vi "niScope EX Multi-Device Configured Acquisition (TClk).vi"() -> ()   [LabVIEW 2013]
doc: "Example: TClk Synchronized Configured Acquisition\n\nRecommended Input Signal: 100 kHz, 4 Vpp, sine wave\n\nDevices Supported: Refer to NI Example Finder\n\nDescription:\n\nThis example configures all the digitizer's vertical, horizontal, and triggering properties before every acquisition. It allows you to experiment with numerous configurations, including acquisition types and triggering modes, since it supports nearly the entire functionality of NI-SCOPE.\n\nThis example also demonstrates how to easily synchronize an arbitrary number of digitizers with niTClk. The niTClk Configure for Homogeneous Triggers, niTClk Synchronize, and niTClk Initiate VIs make this very simple to accomplish. niTClk is useful when synchronized sampling and subsample trigger position are desired. Please refer to the niTClk documentation for more information.\n\nMany parameters are included on the front panel of this example. Notice the \"min sample rate\" compared to the \"actual sample rate,\" and similarly the \"min record length\" to the \"actual record length.\" The \"min\" values are specified with the Configure Horizontal Timing VI. NI-SCOPE maintains a constant time per record for each acquisition. So when you specify a min sample rate and a min record length, this determines the amount of time the acquisition should take:\n\n time per record = min record length / min sampling rate. \n\nHowever, digitizers support only a certain number of defined sampling rates, so if the value chosen is not a valid rate, it is rounded to the next higher rate, called the actual sample rate. The actual record length is then calculated in order to maintain the time per record. Both of these values are returned in this example so you can investigate the effects of parameter rounding with your digitizer. For more information about parameter coercions, see the NI High Speed Digitizers Help.\n\nKeep in mind that not all digitizers support all the features in this example. The NI High Speed Digitizers Help includes a table of supported features for each device."
uses:
  <instrlib>/niScope/Controls/niScope vertical coupling.ctl
  <instrlib>/niScope/Controls/niScope trigger slope.ctl
  <instrlib>/niScope/Controls/niScope polarity.ctl
  <instrlib>/niScope/Controls/niScope tv event.ctl
  <instrlib>/niScope/Controls/niScope trigger coupling.ctl
  <instrlib>/niScope/Controls/niScope trigger window mode.ctl
  <instrlib>/niScope/Controls/niScope trigger source digital.ctl
  <instrlib>/niScope/Controls/niScope signal format.ctl
  <instrlib>/niScope/Controls/niScope trigger source.ctl
  <vilib>/Utility/error.llb/DialogType.ctl
  <instrlib>/niScope/Configure/Trigger/niScope Configure Trigger Edge.vi
  <instrlib>/niScope/Configure/Trigger/niScope Configure Video Trigger.vi
  <instrlib>/niScope/Configure/Trigger/niScope Configure Trigger Hysteresis.vi
  <instrlib>/niScope/Configure/Trigger/niScope Configure Trigger Digital.vi
  <instrlib>/niScope/Configure/Trigger/niScope Configure Trigger Window.vi
  <instrlib>/niScope/Configure/Trigger/niScope Configure Trigger Immediate.vi
  <instrlib>/niScope/Acquire/Fetch/niScope Multi Fetch Cluster.vi
panel:
  in  "Resources":refnum<k15>[](array[refnum])=["Dev1", "Dev2"]
  out "Actual Sample Rate":dbl=10000000.0
  out "Waveform Graph":T1(graph)
  in  "Reference Position (%)":dbl=50.0 caption="Ref Position" format="%.1f"
  in  "Timeout (s)":dbl=5.0 caption="Timeout(s)" format="%.2f"
  in  "Channel Name":string="0" caption="Channel Name(s)"
  in  "Trigger":T2(tab)
  in  "Trigger Source Edge":T3="0" caption="Source"
  in  "Coupling":T4=1 items=["AC"=0, "DC"=1, "HF Reject"=3, "LF Reject"=4, "AC Plus HF Reject"=1001]
  in  "Slope":T5 caption="Trigger Slope"
  in  "Level":dbl caption="Trigger Level" format="%.2f"
  in  "Delay":dbl caption="Trigger Delay" format="%.4p"
  in  "Trigger Source Window":T3="0" caption="Source"
  in  "Window Mode":T6
  in  "Delay":dbl caption="Trigger Delay" format="%.4f"
  in  "Low Level":dbl=-0.1 format="%.2f"
  in  "High Level":dbl=0.1 format="%.2f"
  in  "Window Coupling":T4=1 caption="Coupling" items=["AC"=0, "DC"=1, "HF Reject"=3, "LF Reject"=4, "AC Plus HF Reject"=1001]
  in  "Hysteresis Source Trigger":T3="0" caption="Source"
  in  "Hysteresis":dbl=0.05 format="%.2f"
  in  "Delay":dbl caption="Trigger Delay" format="%.4f"
  in  "Slope":T5 caption="Trigger Slope"
  in  "Hysteresis Coupling":T4=1 caption="Coupling" items=["AC"=0, "DC"=1, "HF Reject"=3, "LF Reject"=4, "AC Plus HF Reject"=1001]
  in  "Level":dbl caption="Trigger Level" format="%.2f"
  in  "Trigger Source Video":T3="0" caption="Source"
  in  "Signal Format":T7=1 caption="signal format" items=["M-NTSC"=1, "B/G-PAL"=2, "SECAM"=3, "M-PAL"=1001, "480i/59.94 fps"=1010, "480i/60 fps"=1011, "480p/59.94 Fps"=1015, "480p/60 Fps"=1016, "576i/50 fps"=1020, "576p/50 Fps"=1025, "720p/50 Fps"=1031, "720p/59.94 Fps"=1032, "720p/60 Fps"=1033, "1080i/50 fps"=1040, "1080i/59.94 fps"=1041, "1080i/60 fps"=1042, "1080p/24 Fps"=1045]
  in  "Trigger Coupling Video":T4=1 caption="Coupling" items=["AC"=0, "DC"=1, "HF Reject"=3, "LF Reject"=4, "AC Plus HF Reject"=1001]
  in  "Delay":dbl caption="Trigger Delay" format="%.4f"
  in  "TV Event":T8=4 items=["Field 1"=1, "Field 2"=2, "Any Field"=3, "Any Line"=4, "Line Number"=5]
  in  "Polarity":T9=2 items=["Positive"=1, "Negative"=2]
  in  "DC Restore":bool
  in  "Line Number":i32=1
  in  "Source":T10="VAL_RTSI_0"
  in  "Delay":dbl caption="Trigger Delay" format="%.4f"
  in  "Slope":T5 caption="Trigger Slope"
  in  "Vertical Coupling":T11=1 items=["AC", "DC", "Ground"]
  in  "Probe Attenuation":dbl=1.0 format="%.1f"
  in  "Vertical Offset":dbl format="%.4f"
  in  "Vertical Range":dbl=10.0 caption="Vertical Range (V)" format="%.2f"
  in  "Bandwidth":dbl=-1.0 format="%.2f"
  in  "Input Impedance":u32(ring) items=["1 mega ohm", "75 ohms", "50 ohms"]
  in  "Min Record Length":i32=1000 caption="Min. Record Length"
  in  "Min Sample Rate":dbl=10000000.0 caption="Min. Sample Rate" step=1000000.0 format="%.2p"
  out "Actual Record Length":i32=1000
  in  "stop":bool
  out "error out":errorcluster={"status"=FALSE, "code"=0, "source"="No Error"} {"code" format="%.0x"}
  # "General"
  # "Horizontal"
  # "Vertical"
  # "Channel"
  # "Trigger"
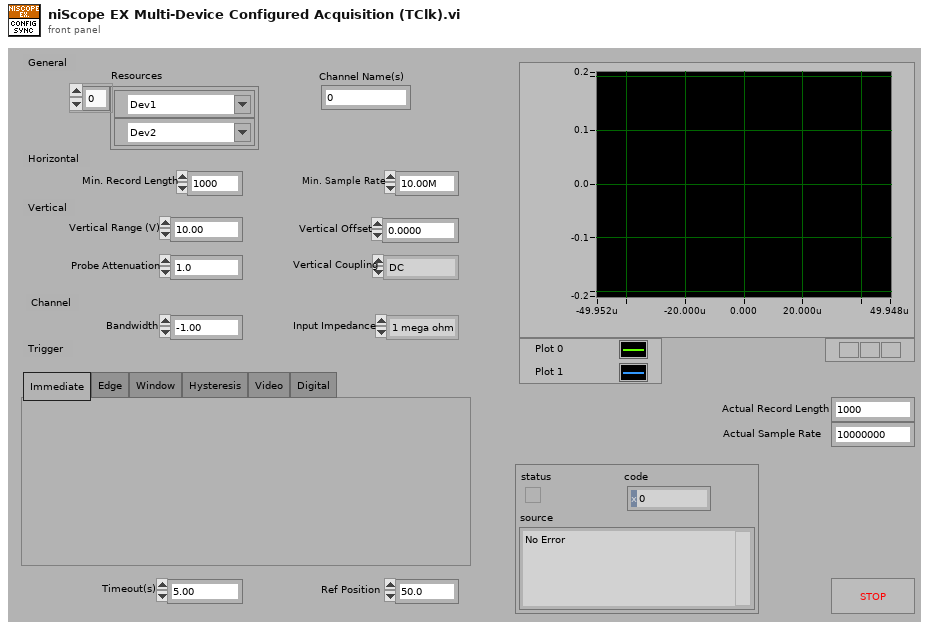
[diagram p1: front panel]
types:
  T1 = cluster{"first point time":dbl, "xIncrement":dbl, "Waveforms":dbl[]}[]
  T2 = enum32{"Immediate", "Edge", "Window", "Hysteresis", "Video", "Digital"}
  T3 = typedef "niScope trigger source.ctl" = string
  T4 = typedef "niScope trigger coupling.ctl" = u16
  T5 = typedef "niScope trigger slope.ctl" = i32
  T6 = typedef "niScope trigger window mode.ctl" = i32
  T7 = typedef "niScope signal format.ctl" = i32
  T8 = typedef "niScope tv event.ctl" = i32
  T9 = typedef "niScope polarity.ctl" = u16
  T10 = typedef "niScope trigger source digital.ctl" = string
  T11 = typedef "niScope vertical coupling.ctl" = i32
  T12 = typedef "DialogType.ctl" = u16
  T13 = cluster{"relativeInitialX":dbl, "xIncrement":dbl, "wfm":dbl[]}[]
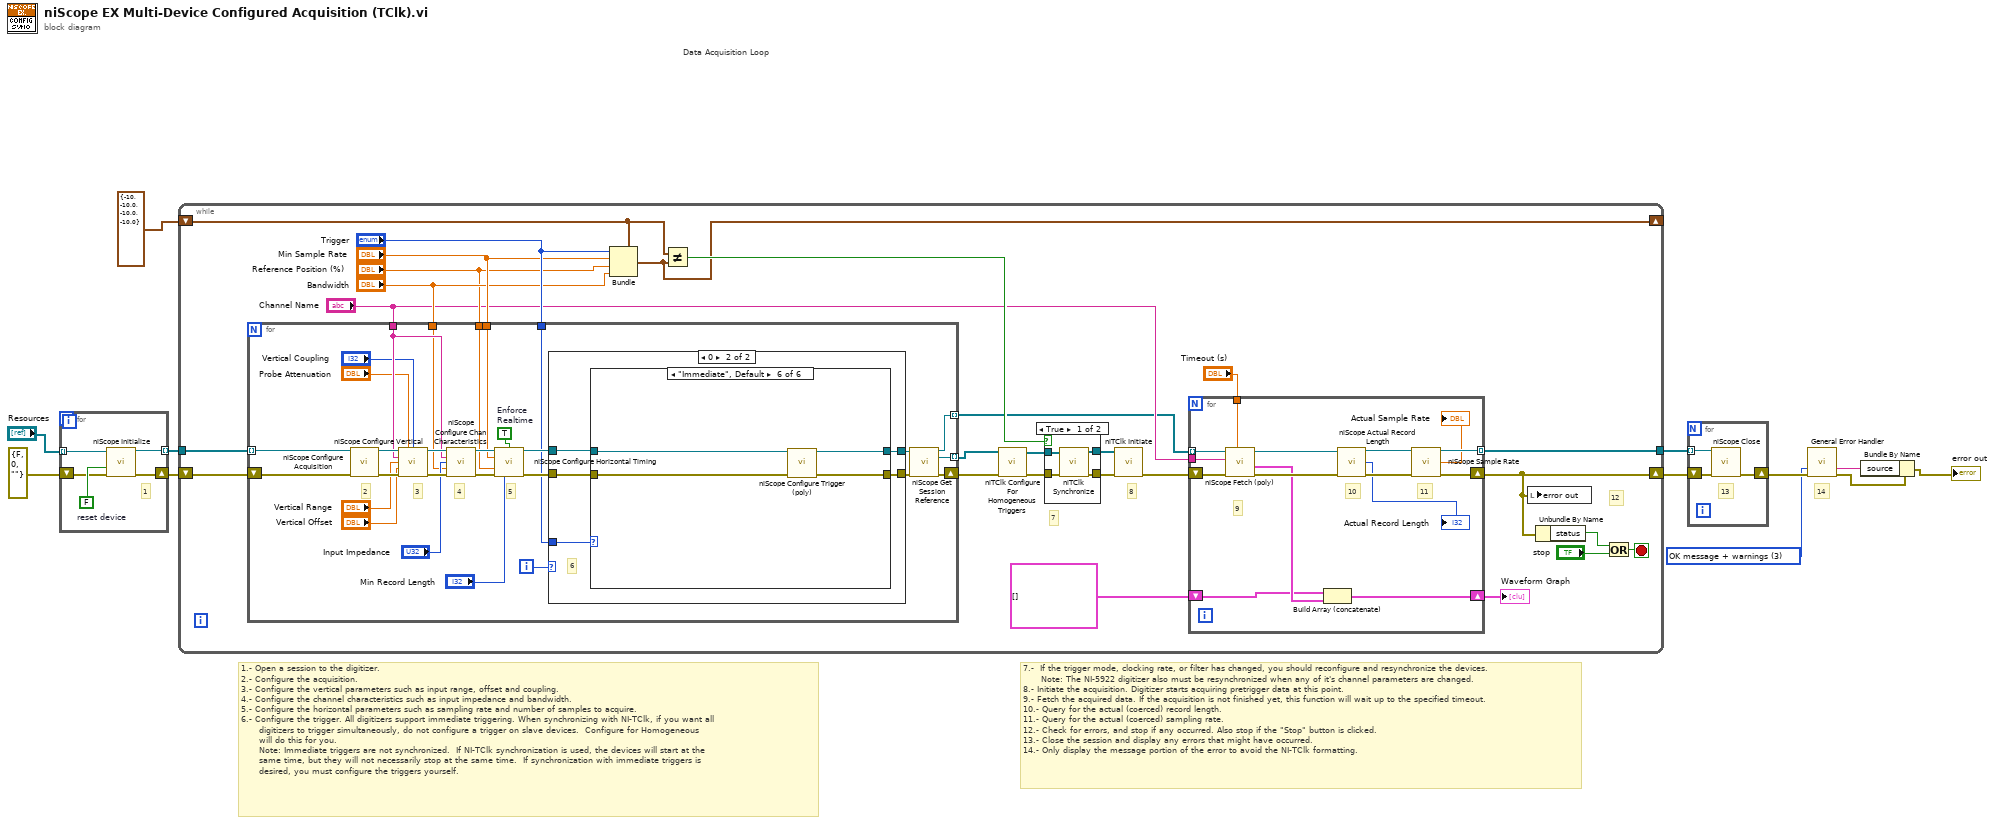
[diagram p0: block diagram]
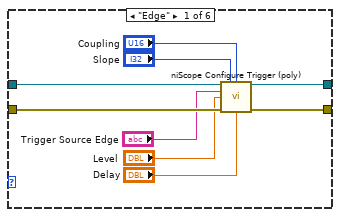
[diagram p4: hidden frame]
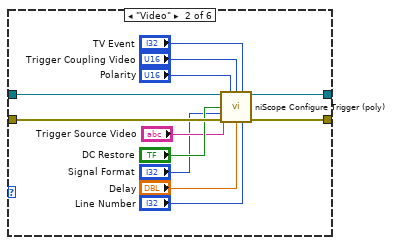
[diagram p5: hidden frame]
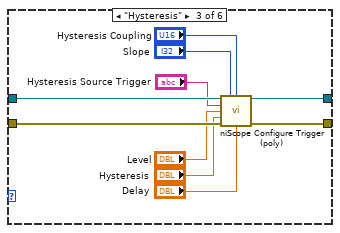
[diagram p6: hidden frame]
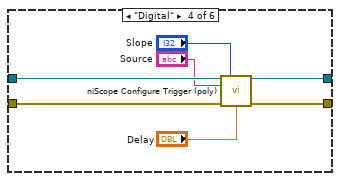
[diagram p7: hidden frame]
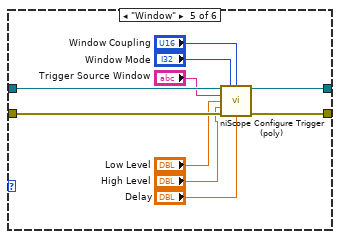
[diagram p8: hidden frame]
diagram:
  w6 = T12 3 items=["no dialog", "OK message", "continue or stop message", "OK message + warnings", "continue/stop + warnings"] ("type of dialog (OK msg:1)")
  # "14"
  # "7.-  If the trigger mode, clocking rate, or filter has changed, you should reconfigure and resynchronize the devices.\n      Note: The NI-5922 digitizer also must be resynchronized when any of it's channel parameters are changed.\n8.- Initiate the acquisition. Digitizer starts acquiring pretrigger data at this point. \n9.- Fetch the acquired data. If the acquisition is not finished yet, this function will wait up to the specified timeout.\n10.- Query for the actual (coerced) record length.\n11.- Query for the actual (coerced) sampling rate.\n12.- Check for errors, and stop if any occurred. Also stop if the \"Stop\" button is clicked.\n13.- Close the session and display any errors that might have occurred.\n14.- Only display the message portion of the error to avoid the NI-TClk formatting."
  # "Data Acquisition Loop"
  # "1.- Open a session to the digitizer.\n2.- Configure the acquisition.\n3.- Configure the vertical parameters such as input range, offset and coupling.\n4.- Configure the channel characteristics such as input impedance and bandwidth.\n5.- Configure the horizontal parameters such as sampling rate and number of samples to acquire.\n6.- Configure the trigger. All digitizers support immediate triggering. When synchronizing with NI-TClk, if you want all\n      digitizers to trigger simultaneously, do not configure a trigger on slave devices.  Configure for Homogeneous\n      will do this for you.\n      Note: Immediate triggers are not synchronized.  If NI-TClk synchronization is used, the devices will start at the\n      same time, but they will not necessarily stop at the same time.  If synchronization with immediate triggers is\n      desired, you must configure the triggers yourself."
  n1 = for {
    tunnel: "Resources" -> [w16] mode=indexing
    tunnel: [w14] -> w9 mode=indexing
    shift-right: [w13] -> w8
    shift-left: errorcluster {"status"=FALSE, "code"=0, "source"=""} ("error out") -> [w15]
    w17 = FALSE  # reset device
    # "1"
    n2 = call <instrlib>:"niScope Initialize.vi"("resource name"=w16, "reset device"=w17, "error in"=w15) -> ("instrument handle"=w14:refnum<k15>, "error out"=w13:errorcluster)  [unwired: 11 in]
  }
  n3 = while {
    shift-right: [w40] -> w11
    shift-left: w8 -> [w42]
    tunnel: w9 -> [w43]
    tunnel: [w41] -> w10
    shift-right: [w27] -> _
    shift-left: cluster{i32, dbl, dbl, dbl} {-10, -10.0, -10.0, -10.0} -> [w28]
    stop <- w35 stop-if-true
    # "8"
    # "7"
    # "12"
    n4 = for {
      tunnel: w43 -> [w77] mode=indexing
      shift-right: [w53] -> w22
      shift-left: w42 -> [w76]
      tunnel: "Channel Name" -> [w67]
      tunnel: "Min Sample Rate" -> [w59]
      tunnel: "Trigger" -> [w58]
      tunnel: "Bandwidth" -> [w56]
      tunnel: "Reference Position (%)" -> [w55]
      tunnel: [w52] -> w19 mode=indexing
      tunnel: [w51] -> w18 mode=indexing
      i -> [w60]
      w74 = TRUE  # Enforce Realtime
      # "2"
      # "3"
      # "4"
      # "5"
      n5 = call <instrlib>:"niScope Configure Acquisition.vi"("instrument handle"=w77, "error in"=w76) -> ("instrument handle out"=w72:refnum<k15>, "error out"=w73:errorcluster)  [unwired: 12 in]
      n6 = call <instrlib>:"niScope Configure Vertical.vi"("instrument handle"=w72, "probe attenuation"="Probe Attenuation", "vertical coupling"="Vertical Coupling", "channels"=w67, "vertical range"="Vertical Range", "vertical offset"="Vertical Offset", "error in"=w73) -> ("instrument handle out"=w71:refnum<k15>, "error out"=w70:errorcluster)  [unwired: 7 in]
      n7 = call <instrlib>:"niScope Configure Chan Characteristics.vi"("instrument handle"=w71, "channels"=w67, "input impedance"="Input Impedance", "maximum input frequency"=w56, "error in"=w70) -> ("instrument handle out"=w68:refnum<k15>, "error out"=w69:errorcluster)  [unwired: 9 in]
      n8 = call <instrlib>:"niScope Configure Horizontal Timing.vi"("instrument handle"=w68, "enforce realtime"=w74, "min sample rate"=w59, "reference position"=w55, "error in"=w69, "min record length"="Min Record Length") -> ("instrument handle out"=w62:refnum<k15>, "error out"=w63:errorcluster)  [unwired: 8 in]
      n9 = case shown="0" w60 {
        tunnel: w63 -> [w78 w84]
        tunnel: w62 -> [w79 w83]
        tunnel: [w79 w82] -> w50
        tunnel: [w78 w81] -> w54
        tunnel: w58 -> [_ w80]
        frame 1, Default {
        }
        frame 0 {
          # "6"
          n10 = case "Trigger Selection" shown="\"Immediate\", Default" w80 {
            tunnel: w84 -> [w93 w105 w115 w122 w132 w136]
            tunnel: [w90 w102 w112 w119 w129 w133] -> w81
            tunnel: w83 -> [w92 w104 w114 w121 w131 w135]
            tunnel: [w91 w103 w113 w120 w130 w134] -> w82
            frame "Edge" {
              n11 = call-poly <instrlib>:"niScope Configure Trigger (poly).vi"("instrument handle"=w92, "trigger slope"="Slope", "trigger coupling"="Coupling", "trigger source"="Trigger Source Edge", "trigger level"="Level", "error in"=w93, "trigger delay"="Delay") -> ("instrument handle out"=w91:refnum<k15>, "error out"=w90:errorcluster)  [unwired: 7 in]
            }
            frame "Video" {
              n12 = call-poly <instrlib>:"niScope Configure Trigger (poly).vi"("instrument handle"=w104, "polarity"="Polarity", "trigger coupling"="Trigger Coupling Video", "TV event"="TV Event", "trigger source"="Trigger Source Video", "enable DC restore"="DC Restore", "signal format"="Signal Format", "error in"=w105, "trigger delay"="Delay", "line number"="Line Number") -> ("instrument handle out"=w103:refnum<k15>, "error out"=w102:errorcluster)  [unwired: 4 in]
            }
            frame "Hysteresis" {
              n13 = call-poly <instrlib>:"niScope Configure Trigger (poly).vi"("instrument handle"=w114, "trigger slope"="Slope", "trigger coupling"="Hysteresis Coupling", "trigger source"="Hysteresis Source Trigger", "trigger level"="Level", "hysteresis"="Hysteresis", "error in"=w115, "trigger delay"="Delay") -> ("instrument handle out"=w113:refnum<k15>, "error out"=w112:errorcluster)  [unwired: 6 in]
            }
            frame "Digital" {
              n14 = call-poly <instrlib>:"niScope Configure Trigger (poly).vi"("instrument handle"=w121, "trigger slope"="Slope", "trigger source"="Source", "error in"=w122, "trigger delay"="Delay") -> ("instrument handle out"=w120:refnum<k15>, "error out"=w119:errorcluster)  [unwired: 9 in]
            }
            frame "Window" {
              n15 = call-poly <instrlib>:"niScope Configure Trigger (poly).vi"("instrument handle"=w131, "trigger window mode"="Window Mode", "trigger coupling"="Window Coupling", "trigger source"="Trigger Source Window", "low level"="Low Level", "high level"="High Level", "error in"=w132, "trigger delay"="Delay") -> ("instrument handle out"=w130:refnum<k15>, "error out"=w129:errorcluster)  [unwired: 6 in]
            }
            frame "Immediate", Default {
              n16 = call-poly <instrlib>:"niScope Configure Trigger (poly).vi"("instrument handle"=w135, "error in"=w136) -> ("instrument handle out"=w134:refnum<k15>, "error out"=w133:errorcluster)  [unwired: 12 in]
            }
          }
        }
      }
      n17 = call <instrlib>:"niScope Get Session Reference.vi"("instrument handle"=w50, "error in"=w54) -> ("instrument handle out"=w52:refnum<k15>, "session reference"=w51:refnum<k20>, "error out"=w53:errorcluster)  [unwired: 11 in]
    }
    n18 = Bundle(cluster=w28, "Trigger", "Min Sample Rate", "Reference Position (%)", "Bandwidth") -> (w27:cluster{i32, dbl, dbl, dbl})
    n19 = Not Equal?(x=w28, y=w27) -> (x != y?=w29:bool)
    n20 = call <instrlib>:"niTClk Configure For Homogeneous Triggers.vi"("error in (no error)"=w22, "sessions"=w18) -> ("error out"=w21:errorcluster, "sessions out"=w20:refnum<k20>[])  [unwired: 8 in]
    n21 = case shown="True" w29 {
      tunnel: [w47 w49] -> w37
      tunnel: [w46 w48] -> w36
      tunnel: w20 -> [w44 w49]
      tunnel: w21 -> [w45 w48]
      frame True {
        n22 = call <instrlib>:"niTClk Synchronize.vi"("error in (no error)"=w45, "sessions"=w44) -> ("error out"=w46:errorcluster, "sessions out"=w47:refnum<k20>[])  [unwired: 8 in]
      }
      frame False {
      }
    }
    n23 = call <instrlib>:"niTClk Initiate.vi"("error in (no error)"=w36, "sessions"=w37) -> ("error out"=w39:errorcluster)  [unwired: 8 in, 1 out]
    n24 = for {
      tunnel: [w151] -> w41 mode=indexing
      tunnel: "Channel Name" -> [w144]
      tunnel: w19 -> [w140] mode=indexing
      tunnel: "Timeout (s)" -> [w138]
      shift-right: [w149] -> w24
      shift-left: T1 [] ("Waveform Graph") -> [w137]
      shift-right: [w150] -> w40
      shift-left: w39 -> [w139]
      # "11"
      # "9"
      # "10"
      n25 = call-poly <instrlib>:"niScope Fetch (poly).vi"("timeout"=w138, "error in"=w139, "channels"=w144, "instrument handle"=w140) -> ("error out"=w142:errorcluster, "waveform"=w141:T13, "instrument handle out"=w143:refnum<k15>)  [unwired: 4 in, 1 out]
      n26 = Build Array (concatenate)(w137, w141) -> (w149:T13)
      n27 = call <instrlib>:"niScope Actual Record Length.vi"("instrument handle"=w143, "error in"=w142) -> ("instrument handle out"=w148:refnum<k15>, "actual record length"=→"Actual Record Length":i32, "error out"=w147:errorcluster)  [unwired: 11 in]
      n28 = call <instrlib>:"niScope Sample Rate.vi"("instrument handle"=w148, "error in"=w147) -> ("instrument handle out"=w151:refnum<k15>, "actual sample rate"=→"Actual Sample Rate":dbl, "error out"=w150:errorcluster)  [unwired: 11 in]
    }
    "Waveform Graph" <- w24
    n29 = local write "error out"(w40) -> ()
    n30 = Unbundle By Name(w40) -> ("status"=w34:bool)
    n31 = Or(x=w34, y="stop") -> (x .or. y?=w35:bool)
  }
  n32 = for {
    tunnel: w10 -> [w152] mode=indexing
    shift-right: [w154] -> w12
    shift-left: w11 -> [w153]
    # "13"
    n33 = call <instrlib>:"niScope Close.vi"("instrument handle"=w152, "error in"=w153) -> ("error out"=w154:errorcluster)  [unwired: 13 in]
  }
  n34 = call <vilib>:"General Error Handler.vi"("type of dialog (OK msg:1)"=w6, "error in (no error)"=w12) -> ("message"=w3:string, "error out"=w5:errorcluster)  [unwired: 9 in, 3 out]
  n35 = Bundle By Name(cluster=w5, "source"=w3) -> (→"error out":errorcluster)
